vi "Close Serial Port.vi"(11 "VISA resource name":refnum<visa-resource-name>) -> ()   [LabVIEW 2020]
panel:
  out "error out":errorcluster
  in  "error in (no error)":errorcluster
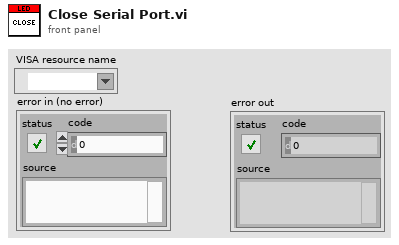
[diagram p1: front panel]
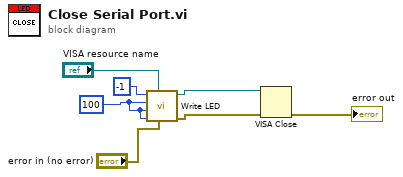
[diagram p0: block diagram]
diagram:
  w2 = u32 100 ("R")
  n1 = call "Write LED.vi"("error in (no error)"="error in (no error)", "VISA resource name"="VISA resource name", "B"=w2, "G"=w2, "R"=w2, "Index"=-1) -> ("error out"=w4:errorcluster, "VISA resource name out"=w1:refnum<visa-resource-name>)  [unwired: 4 in]
  n2 = VISA Close(VISA resource name=w1, error in (no error)=w4) -> (error out=→"error out":errorcluster)
